vi "RunCoordinateSys.vi"(4 "Dllindex":i32, 6 "CreatDllImage":bool, 8 "Error In":errorcluster, 10 "RootPath":path, 11 "Image In":T8(plugin-control)) -> (0 "Error Out":errorcluster, 1 "AnalysisSetting":T1[](array[typedef]) {"ROI"."Contours"."Type" items=["No Selection", "Point", "Line", "Rectangle", "Oval", "Polygon", "Freehand Region", "Annulus", "Unused2", "Unused3", "Broken Line", "Freehand Line", "Rotated Rectangle"]}, 2 "Coordinate System Out":T9 {"Measurement System"."Axis Reference" items=["Direct", "Indirect"]; "Measurement System"."Angle (deg)" format="%.2f"; "Measurement System"."Origin"."Y" format="%.2f"; "Measurement System"."Origin"."X" format="%.2f"; "Reference System"."Axis Reference" items=["Direct", "Indirect"]; "Reference System"."Angle (deg)" format="%.2f"; "Reference System"."Origin"."Y" format="%.2f"; "Reference System"."Origin"."X" format="%.2f"}, 3 "Vision_Image Out":T8(plugin-control), 5 "Main Out":T3[](array[typedef]) {"Analysis_Setting"."Analysis_Type" items=["None", "PatternMatch", "Edge Detection", "Barcode 1D", "Barcode 2D", "Clamp", "Clamp MAX", "Particle", "Histogram", "Straight Edge", "Circle", "Shape Detect", "OCR", "Contour", "ColorMatch"]})   [LabVIEW 2015]
uses:
  Controls/Vision_DataEntry.ctl
  Process/Controls/Process_Setting.ctl
  Process/Controls/Process_Type.ctl
  Analysis/Controls/Analysis_Setting.ctl
  Analysis/Controls/Analysis_Type.ctl
  Control/CoordinateAnalysisSetting.ctl
  Control/CoordinateAction.ctl
  DLL/[Global] Coord.vi
  Analysis/Controls/Parttern Match/Analysis_PatternMatch_ResultWithnumber.ctl
panel:
  out "x-y":u32
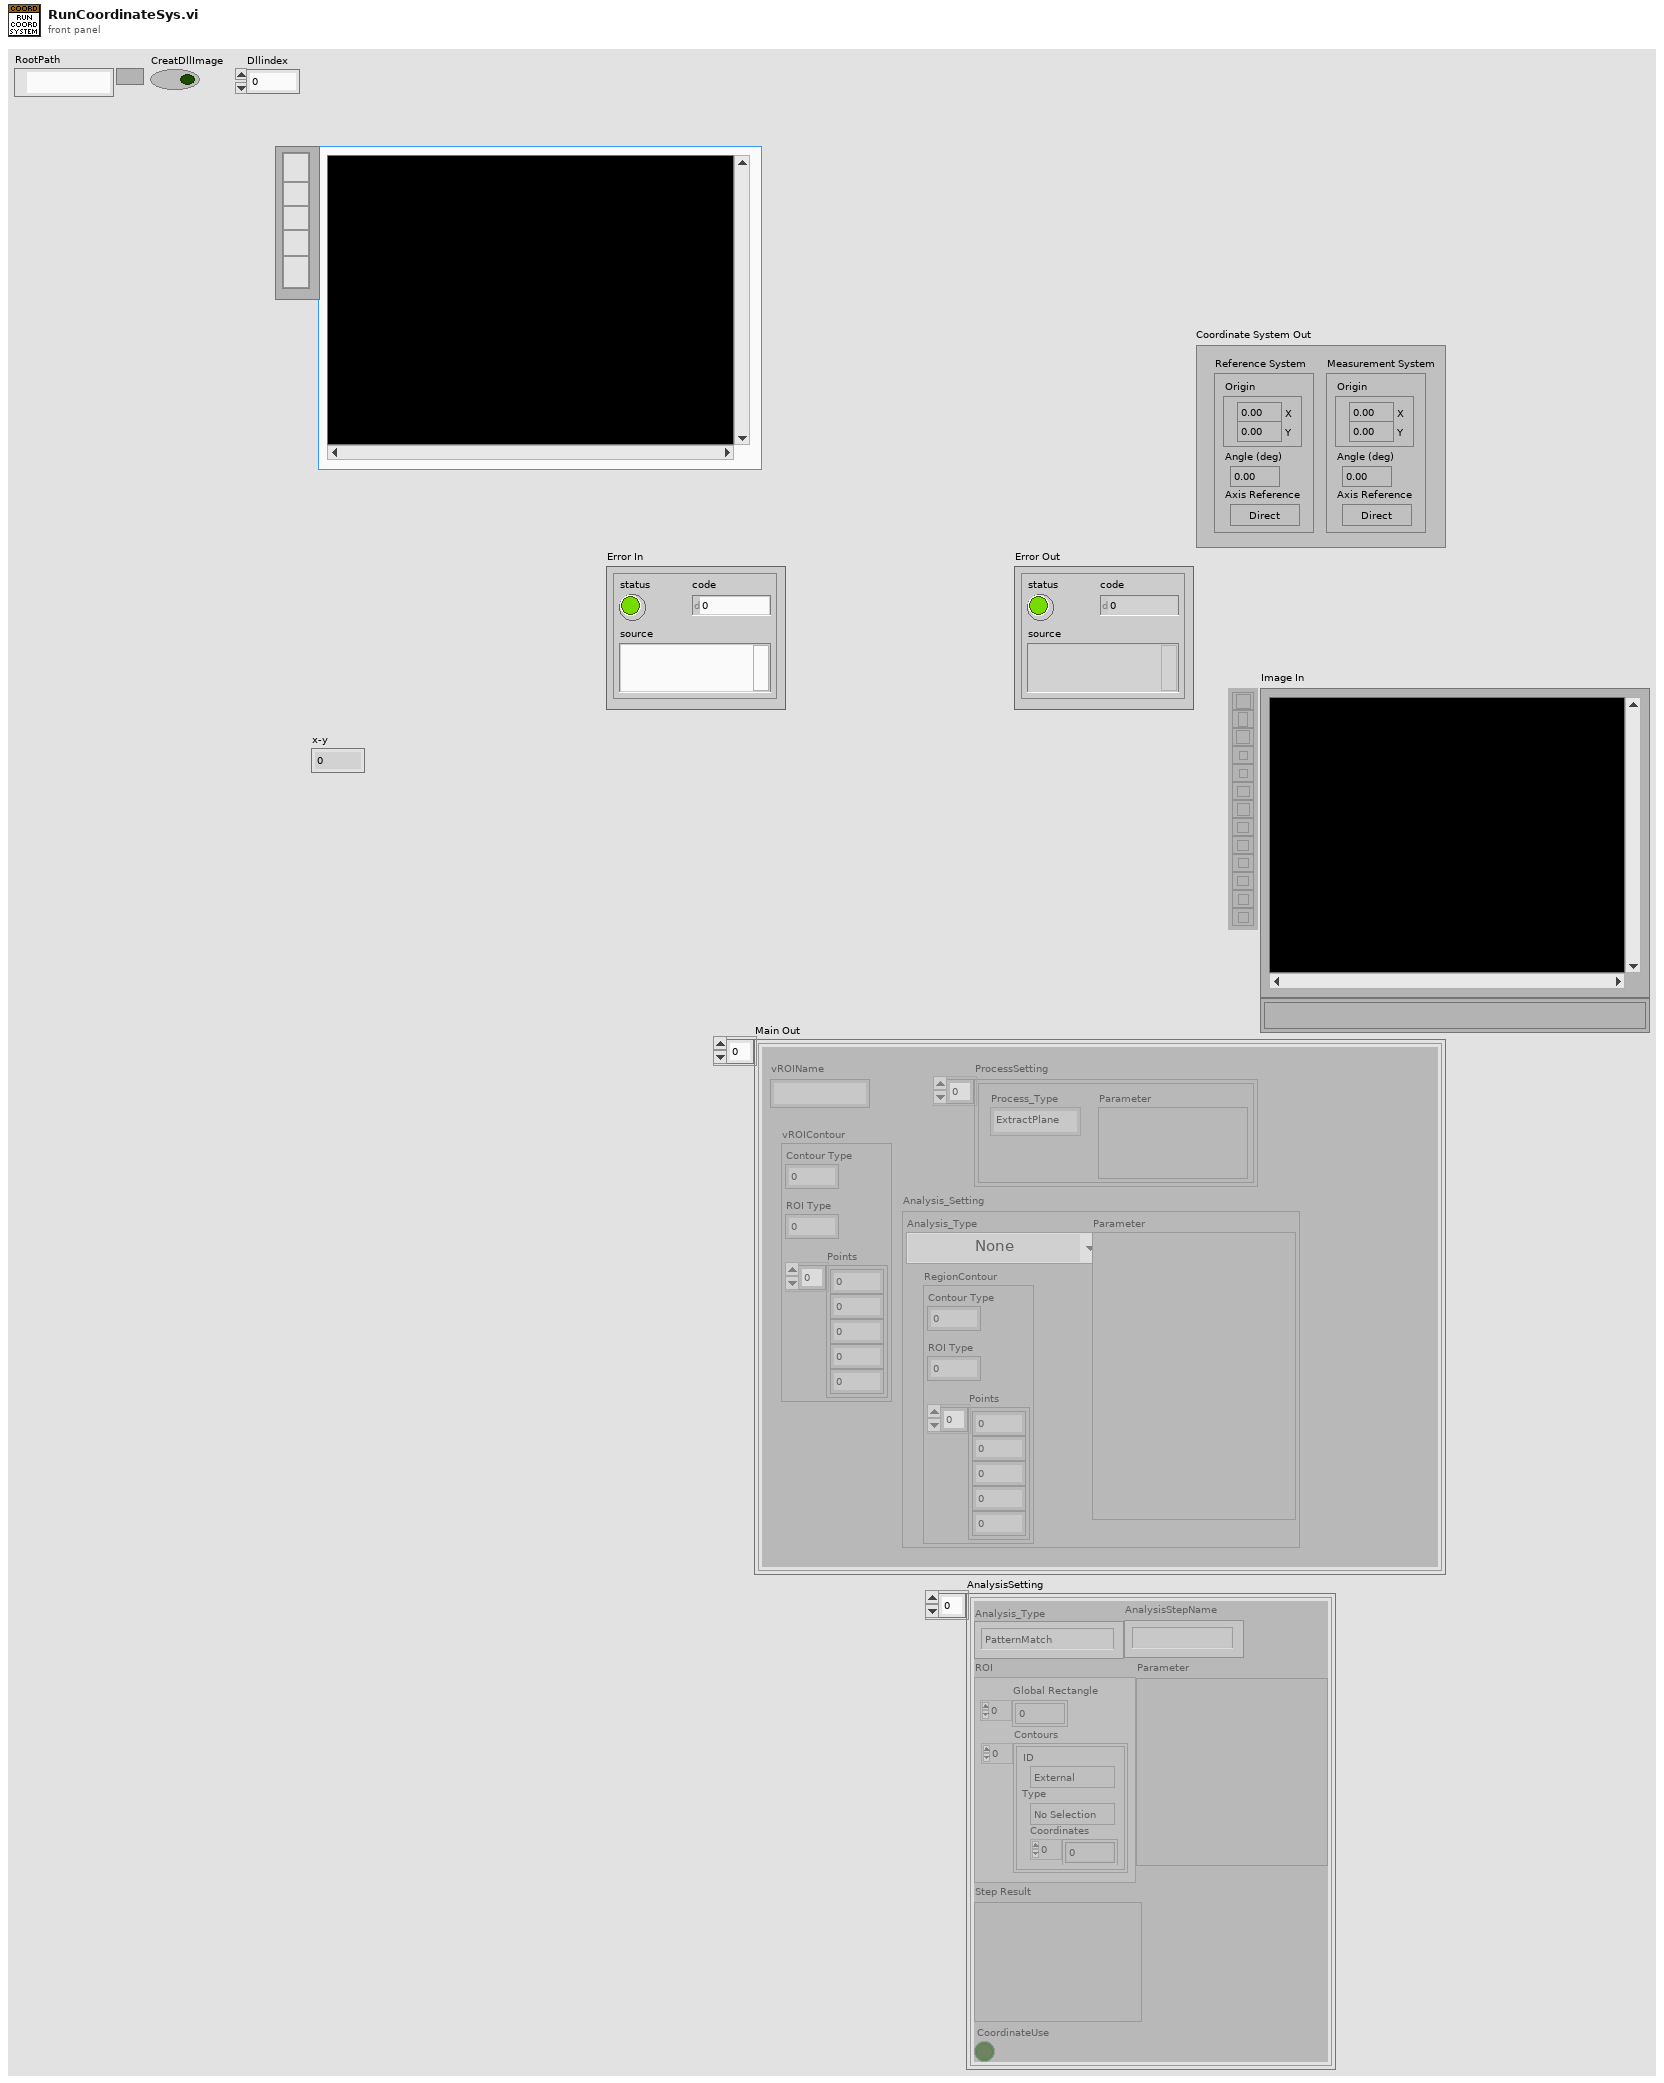
[diagram p1: front panel]
types:
  T1 = typedef "CoordinateAnalysisSetting.ctl" = cluster{"Analysis_Type":enum16{"PatternMatch", "Straight Edge"}, "ROI ":T2, "Parameter":variant, "Step Result":variant, "AnalysisStepName":string, "CoordinateUse":bool}
  T2 = typedef "ROI Descriptor" = cluster{"Global Rectangle":i32[], "Contours":cluster{"ID":enum32{"External", "Internal"}, "Type":u32, "Coordinates":i32[]}[]}
  T3 = typedef "Vision_DataEntry.ctl" = cluster{"vROIName":string, "vROIContour":cluster{"Contour Type":u32, "ROI Type":u32, "Points":i32[]}, "ProcessSetting":T4[], "Analysis_Setting":T6}
  T4 = typedef "Process_Setting.ctl" = cluster{"Process_Type":T5, "Parameter":variant}
  T5 = typedef "Process_Type.ctl" = enum16{"None", "ExtractPlane", "BinaryMono", "Operators", "GrayMorphology", "Filters", "Lookup Table", "Particle Filter", "Mask"}
  T6 = typedef "Analysis_Setting.ctl" = cluster{"Analysis_Type":T7, "RegionContour":cluster{"Contour Type":u32, "ROI Type":u32, "Points":i32[]}, "Parameter":variant}
  T7 = typedef "Analysis_Type.ctl" = u16
  T8 = typedef "IMAQ Image.ctl" = refnum<image>
  T9 = typedef "IMAQ Coordinate System" = cluster{"Reference System":cluster{"Origin":cluster{"X":sgl, "Y":sgl}, "Angle (deg)":sgl, "Axis Reference":u32}, "Measurement System":cluster{"Origin":cluster{"X":sgl, "Y":sgl}, "Angle (deg)":sgl, "Axis Reference":u32}}
  T10 = typedef "CoordinateAction.ctl" = enum16{"Initialize", "CoordEntryInput", "CoordEntryOutput", "CoordEntryTemp", "CoordEntryBackup", "CoordEntryReturn"}
  T11 = typedef "CoordinatteEntry.ctl" = cluster{"ProcessSetting":T4[], "Project Name":string, "AnalysisSetting":T1[], "Coord?":bool, "OriginPointInfo":cluster{"Output Original":bool, "Origin Name":string, "Angle":dbl, "Mode":u16, "OriginPoint":cluster{"X":dbl, "Y":dbl}}, "CaliperSetting":T12[], "CoordIndex":i32[]}
  T12 = typedef "CoordinateCaliperSetting.ctl" = cluster{"Result":variant, "CoordinateUse":bool, "CaliperEntry":T13}
  T13 = typedef "CaliperDataEntry.ctl" = cluster{"CaliperType":T14, "Points":T15[], "Result":T17, "StepName":string}
  T14 = typedef "CaliperType.ctl" = u32
  T15 = typedef "SelectionListEntry.ctl" = cluster{"Type":T16, "Index":i32}
  T16 = typedef "SelectionListEntryPointType.ctl" = enum16{"AnalysisResult", "CaliperResult"}
  T17 = typedef "CaliperResult.ctl" = cluster{"PointInclude?":bool, "Num_Of_Pts":u8, "Position.X":dbl, "Position.Y":dbl, "Angle":dbl, "Distance":dbl, "Area":dbl, "Radius_MAX":dbl, "Radius2_min":dbl, "Dev_Residual":dbl, "P2.X":dbl, "P2.Y":dbl, "StepName":string, "Point ID":u8, "StepError?":bool, "ResultDiff?":bool}
  T18 = typedef "Analysis_PatternMatch_ResultWithnumber.ctl" = cluster{"numbers":i32, "results":cluster{"ROI Descriptor out":T2, "Point":T19, "Angle":sgl, "Score":sgl, "Real World Coordinates":cluster{"X":sgl, "Y":sgl}, "Rectangle":T20}[]}
  T19 = typedef "IMAQ Point" = cluster{"X":sgl, "Y":sgl}
  T20 = typedef "IMAQ Rectangle" = cluster{"Left":i32, "Top":i32, "Right":i32, "Bottom":i32, "Rotation":dbl}
  T21 = cluster{"Point1 (Pixels)":cluster{"X":sgl, "Y":sgl}, "Point2 (Pixels)":cluster{"X":sgl, "Y":sgl}, "Point1 (Real-World)":cluster{"X":sgl, "Y":sgl}, "Point2 (Real-World)":cluster{"X":sgl, "Y":sgl}, "Angle (Pixel)":dbl, "Angle (Real-World)":dbl, "Score":dbl, "Straightness":dbl, "Average SNR (db)":dbl, "Calibration Valid":bool}[]
  T22 = cluster{cluster{void, void, "Axis Reference":u32}, cluster{void, void, "Axis Reference":u32}}
  T23 = cluster{"ROI Descriptor out":T2, "Point":T19, "Angle":sgl, "Score":sgl, "Real World Coordinates":cluster{"X":sgl, "Y":sgl}, "Rectangle":T20}[]
  T24 = cluster{"ROI Descriptor out":T2, "Point":T19, "Angle":sgl, "Score":sgl, "Real World Coordinates":cluster{"X":sgl, "Y":sgl}, "Rectangle":T20}
  T25 = cluster{"Point":T19, "Angle":sgl, "Axis Reference":u32}
  T26 = cluster{"Point1 (Pixels)":cluster{"X":sgl, "Y":sgl}, "Point2 (Pixels)":cluster{"X":sgl, "Y":sgl}, "Point1 (Real-World)":cluster{"X":sgl, "Y":sgl}, "Point2 (Real-World)":cluster{"X":sgl, "Y":sgl}, "Angle (Pixel)":dbl, "Angle (Real-World)":dbl, "Score":dbl, "Straightness":dbl, "Average SNR (db)":dbl, "Calibration Valid":bool}
  T27 = cluster{"Point2 (Pixels)":cluster{"X":sgl, "Y":sgl}, "Angle (Pixel)":dbl, "Axis Reference":u32}
  T28 = cluster{cluster{void, void, "Axis Reference":u32}, cluster{"Point":T19, "Angle (Pixel)":dbl, "Axis Reference":u32}}
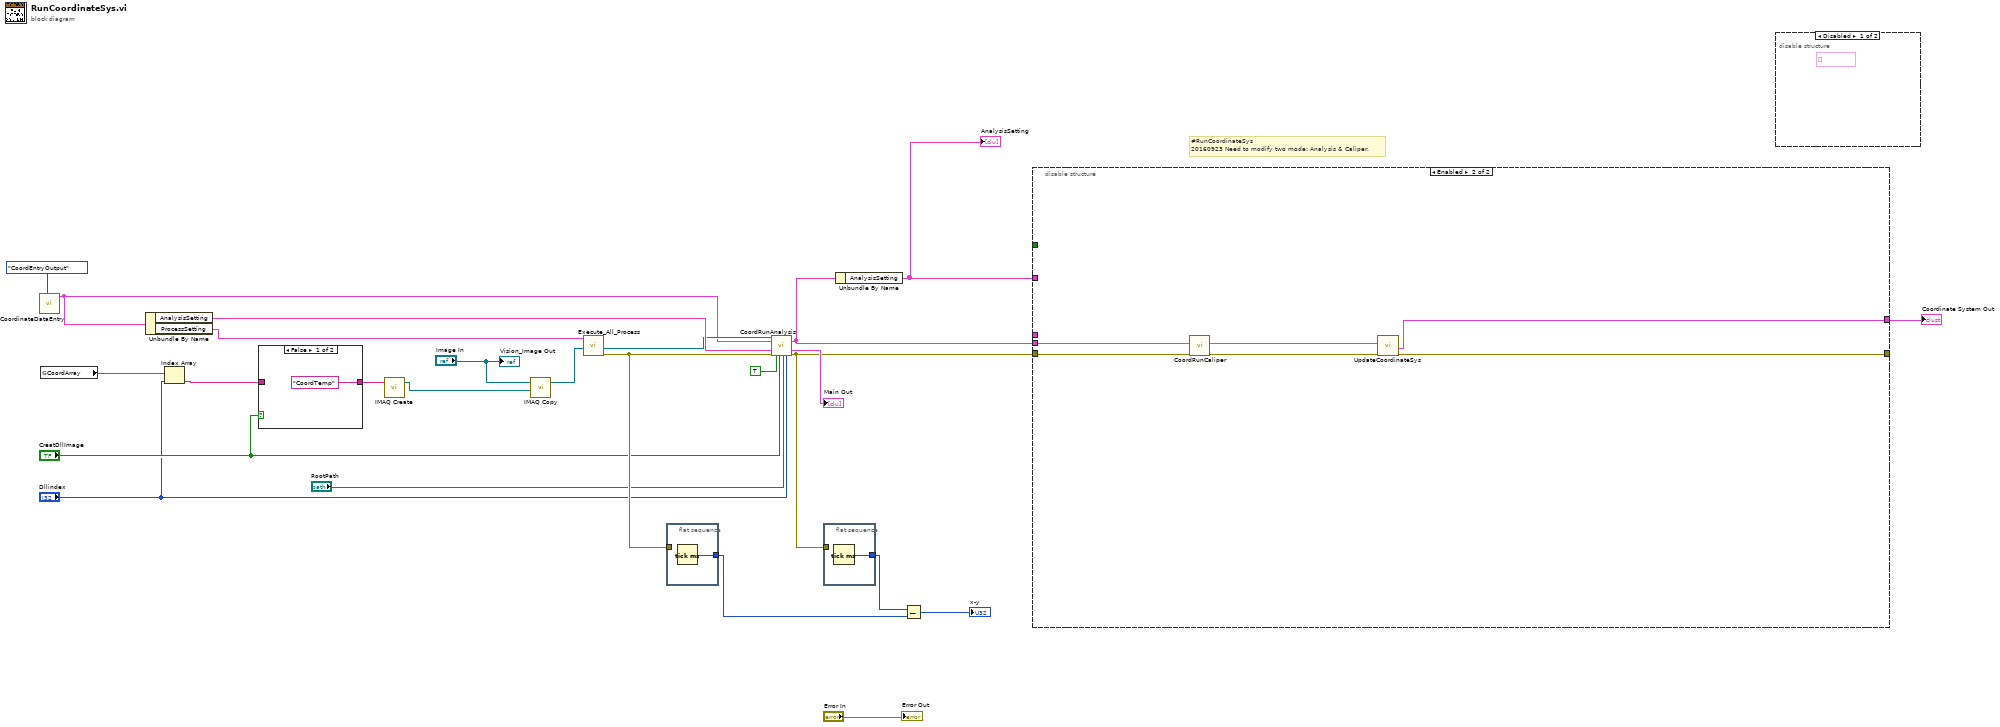
[diagram p0: block diagram]
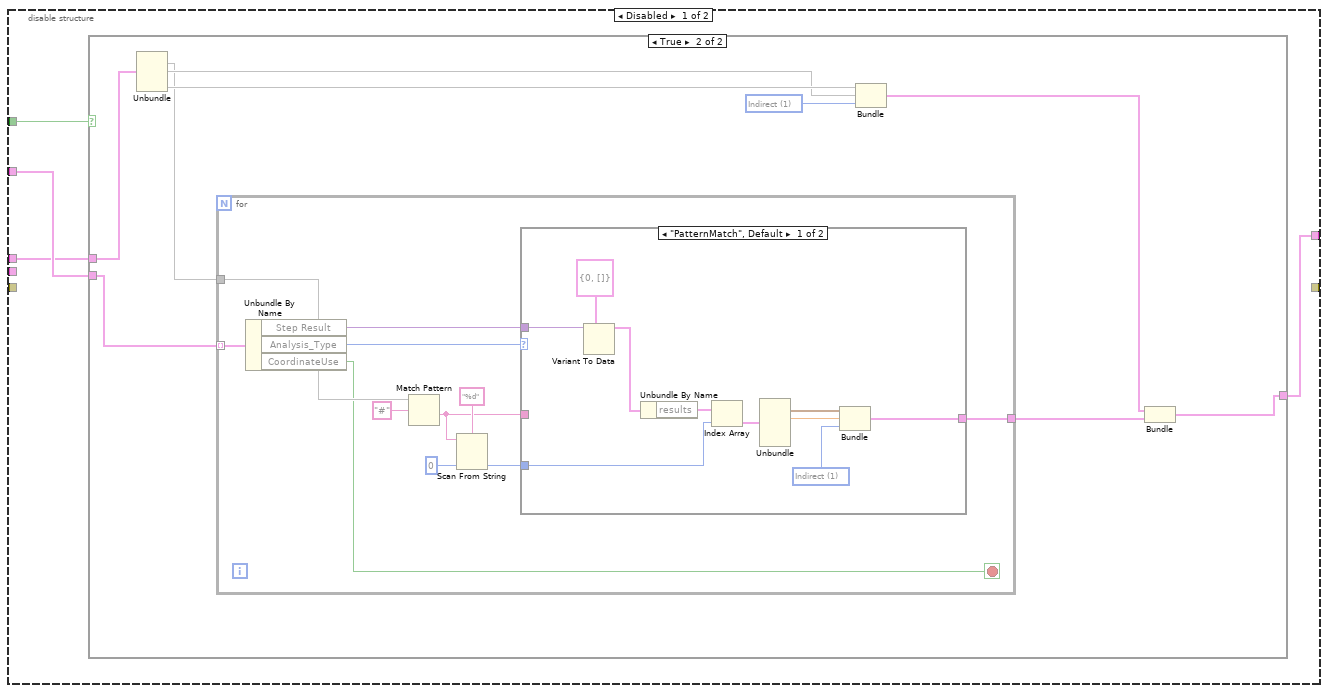
[diagram p2: hidden frame]
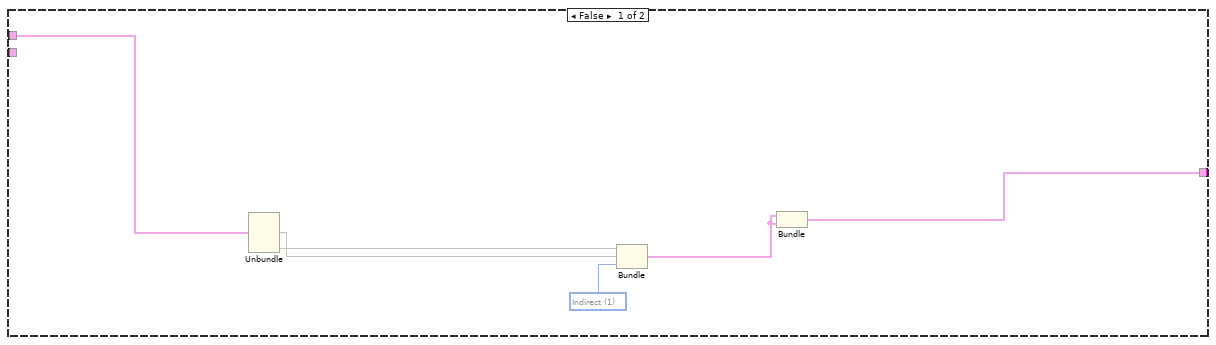
[diagram p3: hidden frame]
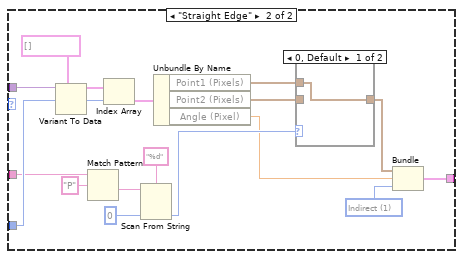
[diagram p4: hidden frame]
diagram:
  # "#RunCoordinateSys\n20160923 Need to modify two mode: Analysis & Caliper."
  n1 = call "CoordinateDataEntry.vi"("CoordinateAction"=CoordinateAction."CoordEntryOutput") -> ("CoordinatteEntry Output"=w16:T11)  [unwired: 9 in, 1 out]
  n2 = global read "[Global] Coord.vi" "CoordArray"() -> (w3:string[])
  n3 = Unbundle By Name(w16) -> ("AnalysisSetting"=w22:T1[], "ProcessSetting"=w23:T4[])
  n4 = Index Array(array=w3, index="Dllindex") -> (element=w8:string)
  n5 = case shown="False" "CreatDllImage" {
    tunnel: ["CoordTemp" ("Image Name") w27] -> w9
    tunnel: w8 -> [_ w27]
    frame False {
    }
    frame True {
    }
  }
  n6 = call "IMAQ Create"("Image Name"=w9) -> ("New Image"=w15:T8)  [unwired: 4 in, 1 out]
  n7 = call "IMAQ Copy"("Image Dst"=w15, "Image Src"="Image In") -> ("Image Dst Out"=w24:T8)  [unwired: 4 in, 1 out]
  n8 = call "Execute_All_Process.vi"("ImageIn"=w24, "ProcessSettingIn"=w23) -> ("error out"=w20:errorcluster, "Image Out"=w21:T8)  [unwired: 4 in, 4 out]
  n9 = flat-sequence {
    tunnel: w20 -> [_]
    tunnel: [w28] -> w18
    frame #0 {
      n10 = Tick Count (ms)() -> (millisecond timer value=w28:u32)
    }
  }
  n11 = call "CoordRunAnalysis.vi"("Refnum in"=w21, "CoordinatteEntry In"=w16, "AnalysisSetting"=w22, "Error In"=w20, "CoordSystemRun?"=TRUE, "CreatDllImage"="CreatDllImage", "RootPath"="RootPath", "Dllindex"="Dllindex") -> ("CoordinatteEntry Out"=w2:T11, "Main Out"=→"Main Out":T3[], "Error Out"=w1:errorcluster)  [unwired: 8 in, 1 out]
  n12 = flat-sequence {
    tunnel: w1 -> [_]
    tunnel: [w29] -> w19
    frame #0 {
      n13 = Tick Count (ms)() -> (millisecond timer value=w29:u32)
    }
  }
  n14 = Unbundle By Name(w2) -> ("AnalysisSetting"=w14:T1[])
  "AnalysisSetting" <- w14
  n15 = Subtract(x=w19, y=w18) -> (x-y=→"x-y":u32)
  n16 = disable-structure shown="Enabled" {
    disable-tunnel: w14 -> [w33 _]
    disable-tunnel: [w32 w94] -> w6
    disable-tunnel: _ -> [w31 _]
    disable-tunnel: _ -> [w30 _]
    disable-tunnel: w2 -> [_ w91]
    disable-tunnel: w1 -> [_ w92]
    disable-tunnel: [_ w93] -> _
    frame Disabled {
      n17 = case shown="True" w31 {
        tunnel: w33 -> [_ w48]
        tunnel: [w34 w41] -> w32
        tunnel: w30 -> [w39 w44]
        frame False {
          w36 = u32 1 items=["Direct", "Indirect"] ("Axis Reference")
          n18 = Unbundle(w39) -> ("Angle"=w37, "OriginPoint"=w38)  [unwired: 3 out]
          n19 = Bundle(w38, w37, "Axis Reference"=w36) -> (w35:cluster{void, void, "Axis Reference":u32})  [unwired: 1 in]
          n20 = Bundle(w35, w35) -> (w34:T22)  [unwired: 1 in]
        }
        frame True {
          w46 = u32 1 items=["Direct", "Indirect"] ("Axis Reference")
          n21 = Unbundle(w44) -> ("Origin Name"=w40, "Angle"=w45, "OriginPoint"=w47)  [unwired: 2 out]
          n22 = for {
            tunnel: w48 -> [w59] mode=indexing
            tunnel: [w51] -> w43
            tunnel: w40 -> [w50]
            stop <- w49 stop-if-true
            n23 = Unbundle By Name(w59) -> ("Step Result"=w52:variant, "Analysis_Type"=w58:enum16{"PatternMatch", "Straight Edge"}, "CoordinateUse"=w49:bool)
            n24 = Match Pattern(string=w50, regular expression="#") -> (after substring=w53:string)  [unwired: 1 in, 3 out]
            n25 = Scan From String(format string="%d", input string=w53, default 1=0) -> (output 1=w54:i32)  [unwired: 2 in, 3 out]
            n26 = case shown="\"PatternMatch\", Default" w58 {
              tunnel: w52 -> [w69 w86]
              tunnel: w54 -> [w68 w82]
              tunnel: [w63 w70] -> w51
              tunnel: w53 -> [_ w80]
              frame "PatternMatch", Default {
                w64 = u32 1 items=["Direct", "Indirect"] ("Axis Reference")
                n27 = Variant To Data(type=T18 {"numbers"=0, "results"=[]} ("PatternMatchResult"), Variant=w69) -> (data=w61:T18)  [unwired: 1 in, 1 out]
                n28 = Unbundle By Name(w61) -> ("results"=w60:T23)
                n29 = Index Array(array=w60, index=w68) -> (element=w67:T24)
                n30 = Unbundle(w67) -> ("Point"=w66:T19, "Angle"=w65:sgl)  [unwired: 4 out]
                n31 = Bundle("Point"=w66, "Angle"=w65, "Axis Reference"=w64) -> (w63:T25)  [unwired: 1 in]
              }
              frame "Straight Edge" {
                w83 = u32 1 items=["Direct", "Indirect"] ("Axis Reference")
                n32 = Variant To Data(type=T21 [], Variant=w86) -> (data=w84:T21)  [unwired: 1 in, 1 out]
                n33 = Match Pattern(string=w80, regular expression="P") -> (after substring=w78:string)  [unwired: 1 in, 3 out]
                n34 = Index Array(array=w84, index=w82) -> (element=w81:T26)
                n35 = Scan From String(format string="%d", input string=w78, default 1=0) -> (output 1=w75:i32)  [unwired: 2 in, 3 out]
                n36 = Unbundle By Name(w81) -> ("Point1 (Pixels)"=w73:cluster{"X":sgl, "Y":sgl}, "Point2 (Pixels)"=w72:cluster{"X":sgl, "Y":sgl}, "Angle (Pixel)"=w71:dbl)
                n37 = case shown="0, Default" w75 {
                  tunnel: [w87 w88] -> w74
                  tunnel: w73 -> [w87 _]
                  tunnel: w72 -> [_ w88]
                  frame 0, Default {
                  }
                  frame 1 {
                  }
                }
                n38 = Bundle("Point2 (Pixels)"=w74, "Angle (Pixel)"=w71, "Axis Reference"=w83) -> (w70:T27)  [unwired: 1 in]
              }
            }
          }
          n39 = Bundle(w47, w45, "Axis Reference"=w46) -> (w42:cluster{void, void, "Axis Reference":u32})  [unwired: 1 in]
          n40 = Bundle(w42, w43) -> (w41:T28)  [unwired: 1 in]
        }
      }
    }
    frame Enabled {
      n41 = call "CoordRunCaliper.vi"("error in (no error)"=w92, "CoordinatteEntry In"=w91) -> ("error out"=w89:errorcluster, "CoordinatteEntry Out"=w90:T11)  [unwired: 8 in]
      n42 = call "UpdateCoordinateSys.vi"("error in (no error)"=w89, "CoordinatteEntry"=w90) -> ("error out"=w93:errorcluster, "Coordinate System Out"=w94:T9)  [unwired: 8 in]
    }
  }
  "Coordinate System Out" <- w6
  n43 = disable-structure shown="Disabled" {
    frame Disabled {
      (unwired) T23 [] ("anything")
    }
    frame Enabled {
    }
  }
  "Error Out" <- "Error In"
  "Vision_Image Out" <- "Image In"
